vi "FGV EPA Leaktest.vi"(6 "Aktion":enum16{"lesen", "schreiben"}(ring), 10 "Leaktest aktiv":u16, 11 "Leaktest Zustand":T1) -> (2 "Leaktest aktiv":bool, 3 "Leaktest Zustand":T1)   [LabVIEW 2020, in "Allgemein.lvlib"]
uses:
  Allgemein.lvlib
  EPA 1065/Dichtheitstest 1065-345/Aktion Leak check durchfuehren.ctl
  EPA 1065/Dichtheitstest 1065-345/Dichtheitstest 1065-345.lvlib
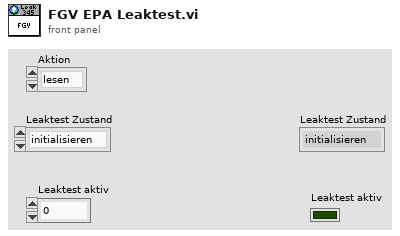
[diagram p1: front panel]
types:
  T1 = typedef "EPA 1065.lvlib/Dichtheitstest 1065-345.lvlib/Aktion Leak check durchfuehren.ctl" = enum16{"initialisieren", "Unterdruck erzeugen", "Ventile schließen", "Warten", "Auswertung", "fertig", "PDF erstellen", "abbrechen"}
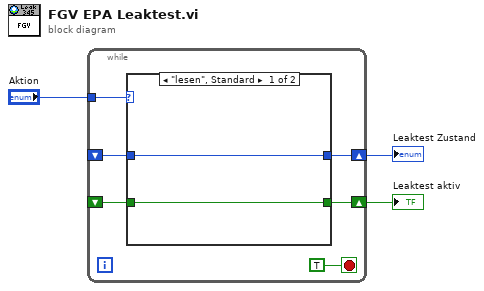
[diagram p0: block diagram]
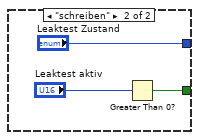
[diagram p2: hidden frame]
diagram:
  n1 = while {
    tunnel: "Aktion" -> [w8]
    shift-right: [w7] -> w2
    shift-left: _ -> [w4]
    shift-right: [w6] -> w1
    shift-left: _ -> [w5]
    stop <- TRUE stop-if-true
    n2 = case shown="\"lesen\", Standard" w8 {
      tunnel: [w11 "Leaktest Zustand"] -> w7
      tunnel: [w10 w12] -> w6
      tunnel: w5 -> [w10 _]
      tunnel: w4 -> [w11 _]
      frame "lesen", Default {
      }
      frame "schreiben" {
        n3 = Greater Than 0?(x="Leaktest aktiv") -> (x > 0?=w12:bool)
      }
    }
  }
  "Leaktest Zustand" <- w2
  "Leaktest aktiv" <- w1
